vi "Get Computer Name.vi"() -> (0 "计算机名称":string)   [LabVIEW 2012]
uses:
  KERNEL32.DLL
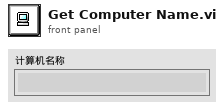
[diagram p1: front panel]
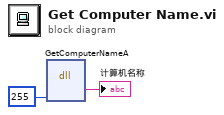
[diagram p0: block diagram]
diagram:
  n1 = dll-call lib="KERNEL32.DLL" fn="GetComputerNameA"("SIZE"=255) -> ("ComputerName"=→"计算机名称":string)  [unwired: 6 in, 2 out]
